vi "Defaults.vi"(8 "error in (no error)":errorcluster, 11 "Formulas in":refnum<class "Formulas Module.lvclass">) -> (0 "error out":errorcluster, 3 "Formulas out":refnum<class "Formulas Module.lvclass">)   [LabVIEW 2021, in "Formulas Module.lvclass"]
uses:
  Formulas Module.lvclass
  C:/Program Files (x86)/National Instruments/LabVIEW 2021/user.lib/S2 Labs/Module Framework/Modules/Formulas/Formulas Base.lvclass
  <userlib>/S2 Labs/Module Framework/Modules/Formulas/TypeDefs/Formula Config Element.ctl
  <userlib>/S2 Labs/Module Framework/Modules/Formulas/Formulas Base.lvclass/Formulas Base.ctl
  <userlib>/S2 Labs/Module Framework/Modules/Formulas/Write Formulas Config.vi
  <userlib>/S2 Labs/Module Framework/Modules/Formulas/Formulas Base.lvclass
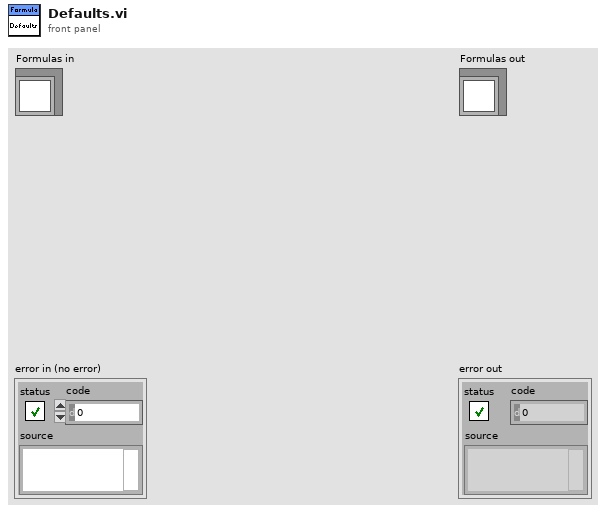
[diagram p1: front panel]
types:
  T1 = typedef "Formulas Base.lvclass/Formula Config Element.ctl" = cluster{"Name":string, "Formula":string, "Unit":string}
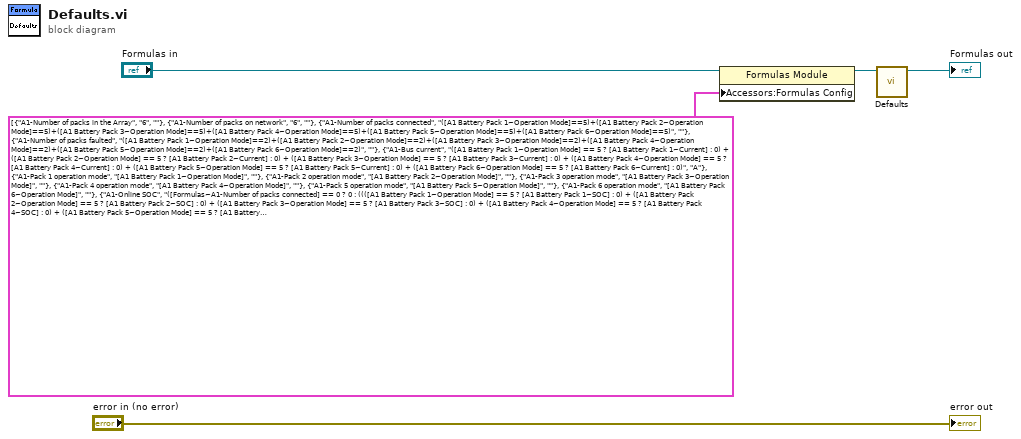
[diagram p0: block diagram]
diagram:
  n1 = property class="Formulas Module"(reference="Formulas in", "Accessors:Formulas Config"=T1[] [{"Name"="A1-Number of packs in the Array", "Formula"="6", "Unit"=""}, {"Name"="A1-Number of packs on network", "Formula"="6", "Unit"=""}, {"Name"="A1-Number of packs connected", "Formula"="([A1 Battery Pack 1~Operation Mode]==5)+([A1 Battery Pack 2~Operation Mode]==5)+([A1 Battery Pack 3~Operation Mode]==5)+([A1 Battery Pack 4~Operation Mode]==5)+([A1 Battery Pack 5~Operation Mode]==5)+([A1 Battery Pack 6~Operation Mode]==5)", "Unit"=""}, {"Name"="A1-Number of packs faulted", "Formula"="([A1 Battery Pack 1~Operation Mode]==2)+([A1 Battery Pack 2~Operation Mode]==2)+([A1 Battery Pack 3~Operation Mode]==2)+([A1 Battery Pack 4~Operation Mode]==2)+([A1 Battery Pack 5~Operation Mode]==2)+([A1 Battery Pack 6~Operation Mode]==2)", "Unit"=""}, {"Name"="A1-Bus current", "Formula"="([A1 Battery Pack 1~Operation Mode] == 5 ? [A1 Battery Pack 1~Current] : 0) + ([A1 Battery Pack 2~Operation Mode] == 5 ? [A1 Battery Pack 2~Current] : 0) + ([A1 Battery Pack 3~Operation Mode] == 5 ? [A1 Battery Pack 3~Current] : 0) + ([A1 Battery Pack 4~Operation Mode] == 5 ? [A1 Battery Pack 4~Current] : 0) + ([A1 Battery Pack 5~Operation Mode] == 5 ? [A1 Battery Pack 5~Current] : 0) + ([A1 Battery Pack 6~Operation Mode] == 5 ? [A1 Battery Pack 6~Current] : 0)", "Unit"="A"}, {"Name"="A1-Pack 1 operation mode", "Formula"="[A1 Battery Pack 1~Operation Mode]", "Unit"=""}, {"Name"="A1-Pack 2 operation mode", "Formula"="[A1 Battery Pack 2~Operation Mode]", "Unit"=""}, {"Name"="A1-Pack 3 operation mode", "Formula"="[A1 Battery Pack 3~Operation Mode]", "Unit"=""}, {"Name"="A1-Pack 4 operation mode", "Formula"="[A1 Battery Pack 4~Operation Mode]", "Unit"=""}, {"Name"="A1-Pack 5 operation mode", "Formula"="[A1 Battery Pack 5~Operation Mode]", "Unit"=""}, {"Name"="A1-Pack 6 operation mode", "Formula"="[A1 Battery Pack 6~Operation Mode]", "Unit"=""}, {"Name"="A1-Online SOC", "Formula"="([Formulas~A1-Number of packs connected] == 0 ? 0 : ((([A1 Battery Pack 1~Operation Mode] == 5 ? [A1 Battery Pack 1~SOC] : 0) + ([A1 Battery Pack 2~Operation Mode] == 5 ? [A1 Battery Pack 2~SOC] : 0) + ([A1 Battery Pack 3~Operation Mode] == 5 ? [A1 Battery Pack 3~SOC] : 0) + ([A1 Battery Pack 4~Operation Mode] == 5 ? [A1 Battery Pack 4~SOC] : 0) + ([A1 Battery Pack 5~Operation Mode] == 5 ? [A1 Battery Pack 5~SOC] : 0) + ([A1 Battery Pack 6~Operation Mode] == 5 ? [A1 Battery Pack 6~SOC] : 0))/[Formulas~A1-Number of packs connected]))", "Unit"="%"}, {"Name"="A1-Online SOH", "Formula"="([Formulas~A1-Number of packs connected] == 0 ? 0 : ((([A1 Battery Pack 1~Operation Mode] == 5 ? [A1 Battery Pack 1~SOH] : 0) + ([A1 Battery Pack 2~Operation Mode] == 5 ? [A1 Battery Pack 2~SOH] : 0) + ([A1 Battery Pack 3~Operation Mode] == 5 ? [A1 Battery Pack 3~SOH] : 0) + ([A1 Battery Pack 4~Operation Mode] == 5 ? [A1 Battery Pack 4~SOH] : 0) + ([A1 Battery Pack 5~Operation Mode] == 5 ? [A1 Battery Pack 5~SOH] : 0) + ([A1 Battery Pack 6~Operation Mode] == 5 ? [A1 Battery Pack 6~SOH] : 0))/[Formulas~A1-Number of packs connected]))", "Unit"="%"}, {"Name"="A1-Bus voltage", "Formula"="([Formulas~A1-Number of packs connected] == 0 ? 0 : ((([A1 Battery Pack 1~Operation Mode] == 5 ? [A1 Battery Pack 1~Bus voltage] : 0) + ([A1 Battery Pack 2~Operation Mode] == 5 ? [A1 Battery Pack 2~Bus voltage] : 0) + ([A1 Battery Pack 3~Operation Mode] == 5 ? [A1 Battery Pack 3~Bus voltage] : 0) + ([A1 Battery Pack 4~Operation Mode] == 5 ? [A1 Battery Pack 4~Bus voltage] : 0) + ([A1 Battery Pack 5~Operation Mode] == 5 ? [A1 Battery Pack 5~Bus voltage] : 0) + ([A1 Battery Pack 6~Operation Mode] == 5 ? [A1 Battery Pack 6~Bus voltage] : 0))/[Formulas~A1-Number of packs connected]))", "Unit"="V"}, {"Name"="A1-Max Online Cell Temp", "Formula"="max(([A1 Battery Pack 1~Operation Mode] == 5 ? [A1 Battery Pack 1~Maximum cell temperature] : 0),([A1 Battery Pack 2~Operation Mode] == 5 ? [A1 Battery Pack 2~Maximum cell temperature] : 0),([A1 Battery Pack 3~Operation Mode] == 5 ? [A1 Battery Pack 3~Maximum cell temperature] : 0),([A1 Battery Pack 4~Operation Mode] == 5 ? [A1 Battery Pack 4~Maximum cell temperature] : 0),([A1 Battery Pack 5~Operation Mode] == 5 ? [A1 Battery Pack 5~Maximum cell temperature] : 0),([A1 Battery Pack 6~Operation Mode] == 5 ? [A1 Battery Pack 6~Maximum cell temperature] : 0))", "Unit"="C"}, {"Name"="A1-System Charge Current Limit", "Formula"="([A1 Battery Pack 1~Operation Mode] == 5 ? [A1 Battery Pack 1~Charge current limit] : 0) + ([A1 Battery Pack 2~Operation Mode] == 5 ? [A1 Battery Pack 2~Charge current limit] : 0) + ([A1 Battery Pack 3~Operation Mode] == 5 ? [A1 Battery Pack 3~Charge current limit] : 0) + ([A1 Battery Pack 4~Operation Mode] == 5 ? [A1 Battery Pack 4~Charge current limit] : 0) + ([A1 Battery Pack 5~Operation Mode] == 5 ? [A1 Battery Pack 5~Charge current limit] : 0) + ([A1 Battery Pack 6~Operation Mode] == 5 ? [A1 Battery Pack 6~Charge current limit] : 0)", "Unit"="A"}, {"Name"="A1-System Discharge Current Limit", "Formula"="([A1 Battery Pack 1~Operation Mode] == 5 ? [A1 Battery Pack 1~Discharge current limit] : 0) + ([A1 Battery Pack 2~Operation Mode] == 5 ? [A1 Battery Pack 2~Discharge current limit] : 0) + ([A1 Battery Pack 3~Operation Mode] == 5 ? [A1 Battery Pack 3~Discharge current limit] : 0) + ([A1 Battery Pack 4~Operation Mode] == 5 ? [A1 Battery Pack 4~Discharge current limit] : 0) + ([A1 Battery Pack 5~Operation Mode] == 5 ? [A1 Battery Pack 5~Discharge current limit] : 0) + ([A1 Battery Pack 6~Operation Mode] == 5 ? [A1 Battery Pack 6~Discharge current limit] : 0)", "Unit"="A"}, {"Name"="A2-Number of packs in the Array", "Formula"="6", "Unit"=""}, {"Name"="A2-Number of packs on network", "Formula"="6", "Unit"=""}, {"Name"="A2-Number of packs connected", "Formula"="([A2 Battery Pack 1~Operation Mode]==5)+([A2 Battery Pack 2~Operation Mode]==5)+([A2 Battery Pack 3~Operation Mode]==5)+([A2 Battery Pack 4~Operation Mode]==5)+([A2 Battery Pack 5~Operation Mode]==5)+([A2 Battery Pack 6~Operation Mode]==5)", "Unit"=""}, {"Name"="A2-Number of packs faulted", "Formula"="([A2Battery Pack 1~Operation Mode]==2)+([A2 Battery Pack 2~Operation Mode]==2)+([A2 Battery Pack 3~Operation Mode]==2)+([A2 Battery Pack 4~Operation Mode]==2)+([A2 Battery Pack 5~Operation Mode]==2)+([A2 Battery Pack 6~Operation Mode]==2)", "Unit"=""}, {"Name"="A2-Bus current", "Formula"="([A2 Battery Pack 1~Operation Mode] == 5 ? [A2 Battery Pack 1~Current] : 0) + ([A2 Battery Pack 2~Operation Mode] == 5 ? [A2 Battery Pack 2~Current] : 0) + ([A2 Battery Pack 3~Operation Mode] == 5 ? [A2 Battery Pack 3~Current] : 0) + ([A2 Battery Pack 4~Operation Mode] == 5 ? [A2 Battery Pack 4~Current] : 0) + ([A2 Battery Pack 5~Operation Mode] == 5 ? [A2 Battery Pack 5~Current] : 0) + ([A2 Battery Pack 6~Operation Mode] == 5 ? [A2 Battery Pack 6~Current] : 0)", "Unit"="A"}, {"Name"="A2-Pack 1 operation mode", "Formula"="[A2 Battery Pack 1~Operation Mode]", "Unit"=""}, {"Name"="A2-Pack 2 operation mode", "Formula"="[A2 Battery Pack 2~Operation Mode]", "Unit"=""}, {"Name"="A2-Pack 3 operation mode", "Formula"="[A2 Battery Pack 3~Operation Mode]", "Unit"=""}, {"Name"="A2-Pack 4 operation mode", "Formula"="[A2 Battery Pack 4~Operation Mode]", "Unit"=""}, {"Name"="A2-Pack 5 operation mode", "Formula"="[A2 Battery Pack 5~Operation Mode]", "Unit"=""}, {"Name"="A2-Pack 6 operation mode", "Formula"="[A2 Battery Pack 6~Operation Mode]", "Unit"=""}, {"Name"="A2-Online SOC", "Formula"="([Formulas~A2-Number of packs connected] == 0 ? 0 : ((([A2 Battery Pack 1~Operation Mode] == 5 ? [A2 Battery Pack 1~SOC] : 0) + ([A2 Battery Pack 2~Operation Mode] == 5 ? [A2 Battery Pack 2~SOC] : 0) + ([A2 Battery Pack 3~Operation Mode] == 5 ? [A2 Battery Pack 3~SOC] : 0) + ([A2 Battery Pack 4~Operation Mode] == 5 ? [A2 Battery Pack 4~SOC] : 0) + ([A2 Battery Pack 5~Operation Mode] == 5 ? [A2 Battery Pack 5~SOC] : 0) + ([A2 Battery Pack 6~Operation Mode] == 5 ? [A2 Battery Pack 6~SOC] : 0))/[Formulas~A2-Number of packs connected]))", "Unit"="%"}, {"Name"="A2-Online SOH", "Formula"="([Formulas~A2-Number of packs connected] == 0 ? 0 : ((([A2 Battery Pack 1~Operation Mode] == 5 ? [A2 Battery Pack 1~SOH] : 0) + ([A2 Battery Pack 2~Operation Mode] == 5 ? [A2 Battery Pack 2~SOH] : 0) + ([A2 Battery Pack 3~Operation Mode] == 5 ? [A2 Battery Pack 3~SOH] : 0) + ([A2 Battery Pack 4~Operation Mode] == 5 ? [A2 Battery Pack 4~SOH] : 0) + ([A2 Battery Pack 5~Operation Mode] == 5 ? [A2 Battery Pack 5~SOH] : 0) + ([A2 Battery Pack 6~Operation Mode] == 5 ? [A2 Battery Pack 6~SOH] : 0))/[Formulas~A2-Number of packs connected]))", "Unit"="%"}, {"Name"="A2-Bus voltage", "Formula"="([Formulas~A2-Number of packs connected] == 0 ? 0 : ((([A2 Battery Pack 1~Operation Mode] == 5 ? [A2 Battery Pack 1~Bus voltage] : 0) + ([A2 Battery Pack 2~Operation Mode] == 5 ? [A2 Battery Pack 2~Bus voltage] : 0) + ([A2 Battery Pack 3~Operation Mode] == 5 ? [A2 Battery Pack 3~Bus voltage] : 0) + ([A2 Battery Pack 4~Operation Mode] == 5 ? [A2 Battery Pack 4~Bus voltage] : 0) + ([A2 Battery Pack 5~Operation Mode] == 5 ? [A2 Battery Pack 5~Bus voltage] : 0) + ([A2 Battery Pack 6~Operation Mode] == 5 ? [A2 Battery Pack 6~Bus voltage] : 0))/[Formulas~A2-Number of packs connected]))", "Unit"="V"}, {"Name"="A2-Max Online Cell Temp", "Formula"="max(([A2 Battery Pack 1~Operation Mode] == 5 ? [A2 Battery Pack 1~Maximum cell temperature] : 0),([A2 Battery Pack 2~Operation Mode] == 5 ? [A2 Battery Pack 2~Maximum cell temperature] : 0),([A2 Battery Pack 3~Operation Mode] == 5 ? [A2 Battery Pack 3~Maximum cell temperature] : 0),([A2 Battery Pack 4~Operation Mode] == 5 ? [A2 Battery Pack 4~Maximum cell temperature] : 0),([A2 Battery Pack 5~Operation Mode] == 5 ? [A2 Battery Pack 5~Maximum cell temperature] : 0),([A2 Battery Pack 6~Operation Mode] == 5 ? [A2 Battery Pack 6~Maximum cell temperature] : 0))", "Unit"="C"}, {"Name"="A2-System Charge Current Limit", "Formula"="([A2 Battery Pack 1~Operation Mode] == 5 ? [A2 Battery Pack 1~Charge current limit] : 0) + ([A2 Battery Pack 2~Operation Mode] == 5 ? [A2 Battery Pack 2~Charge current limit] : 0) + ([A2 Battery Pack 3~Operation Mode] == 5 ? [A2 Battery Pack 3~Charge current limit] : 0) + ([A2 Battery Pack 4~Operation Mode] == 5 ? [A2 Battery Pack 4~Charge current limit] : 0) + ([A2 Battery Pack 5~Operation Mode] == 5 ? [A2 Battery Pack 5~Charge current limit] : 0) + ([A2 Battery Pack 6~Operation Mode] == 5 ? [A2 Battery Pack 6~Charge current limit] : 0)", "Unit"="A"}, {"Name"="A2-System Discharge Current Limit", "Formula"="([A2 Battery Pack 1~Operation Mode] == 5 ? [A2 Battery Pack 1~Discharge current limit] : 0) + ([A2 Battery Pack 2~Operation Mode] == 5 ? [A2 Battery Pack 2~Discharge current limit] : 0) + ([A2 Battery Pack 3~Operation Mode] == 5 ? [A2 Battery Pack 3~Discharge current limit] : 0) + ([A2 Battery Pack 4~Operation Mode] == 5 ? [A2 Battery Pack 4~Discharge current limit] : 0) + ([A2 Battery Pack 5~Operation Mode] == 5 ? [A2 Battery Pack 5~Discharge current limit] : 0) + ([A2 Battery Pack 6~Operation Mode] == 5 ? [A2 Battery Pack 6~Discharge current limit] : 0)", "Unit"="A"}] ("Formulas Config")) -> (reference out=w2:refnum<class "Formulas Module.lvclass">)  [unwired: 1 in, 1 out]
  n2 = call-parent "Defaults.vi"("Formulas in"=w2) -> ("Formulas out"=→"Formulas out":refnum<class "Formulas Module.lvclass">)  [unwired: 9 in, 1 out]
  "error out" <- "error in (no error)"
